vi "Deadband.vi"(1 "Limit":dbl=0.1, 2 "Input":dbl) -> (0 "Output":dbl)   [LabVIEW 2020]
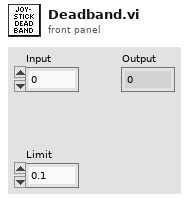
[diagram p1: front panel]
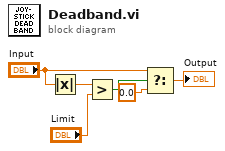
[diagram p0: block diagram]
diagram:
  n1 = Absolute Value(x="Input") -> (abs(x)=w1:dbl)
  n2 = Greater?(x=w1, y="Limit") -> (0:w4:bool)
  n3 = Select(t="Input", s=w4, f=0.0) -> (s? t:f=→"Output":dbl)
